vi "dscDIOOutputByte.vi"(8 "error in":errorcluster, 9 "dig_val":u8, 10 "port":u8, 11 "board":i16) -> (0 "error out":errorcluster, 3 "boardOut":i16)   [LabVIEW 2011, in "Diamond Universal Driver.lvlib"]
doc: "Send a BYTE to a given digital output port."
uses:
  Diamond Universal Driver.lvlib
  Controls/error codes.ctl
  Instruments/WL OPC/Support/dlls/dscud.dll
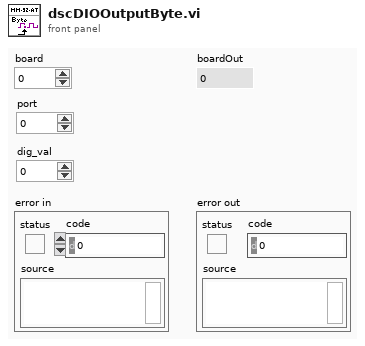
[diagram p1: front panel]
types:
  T1 = typedef "Diamond Universal Driver.lvlib/error codes.ctl" = enum8{"DE_NONE", "DE_HW_FAILURE", "DE_SW_FAILURE", "DE_HW_NOT_SUPPORTED", "DE_SW_NOT_SUPPORTED", "DE_INVALID_PARM", "DE_ALTERNATE_IN_PROGRESS", "DE_NONE_IN_PROGRESS", "DE_BUFFER_ROLLOVER", "DE_INVALID_ERROR_CODE", "DE_ALREADY_PAUSED", "DE_OVERFLOW", "DE_INVALID_FUNC", "DE_DSCUDH_INVALID", "DE_INVALID_BOARD", "DE_BOARD_LIMIT_REACHED", "DE_BOARD_BUSY", "DE_INVALID_WINDRVR_HANDLE", "DE_INVALID_WINDRVR_VERSION", "DE_BAD_WINDRVR_BOARD_INIT", "DE_OPERATION_TIMED_OUT", "DE_INVALID_WINDRVR_KP", "DE_THREAD_FAILURE"}
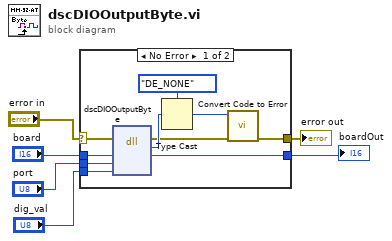
[diagram p0: block diagram]
diagram:
  n1 = case shown="No Error" "error in" {
    selector: "error in" -> [w13 w18]
    tunnel: "board" -> [w11 w17]
    tunnel: [w10 w17] -> w4
    tunnel: [w9 w18] -> w3
    tunnel: "port" -> [w8 _]
    tunnel: "dig_val" -> [w7 _]
    frame No Error {
      n2 = dll-call lib="C:/Users/mrichardson/Documents/Web Based Version Control SW/Instruments/WL OPC/Support/dlls/dscud.dll" fn="dscDIOOutputByte"(error in=w13, "board"=w11, "port"=w8, "dig_val"=w7) -> (error out=w12:errorcluster, "error"=w14:u8, "board"=w10:i16)  [unwired: 4 in, 1 out]
      n3 = Type Cast(type=error_codes."DE_NONE" ("error codes"), x=w14) -> (*(type *) &x=w16:T1)
      n4 = call "Convert Code to Error.vi"("error in"=w12, "error codes"=w16) -> ("error out"=w9:errorcluster)  [unwired: 9 in]
    }
    frame Error {
    }
  }
  "boardOut" <- w4
  "error out" <- w3
